vi "InitConfigParams.vi"(8 "error in (no error)":errorcluster, 10 "configuration file path":path, 11 "Camera in":refnum<class "CameraI2COUSB.lvclass">) -> (0 "error out":errorcluster, 3 "Camera out":refnum<class "CameraI2COUSB.lvclass">)   [LabVIEW 2020, in "CameraI2COUSB.lvlib" / "CameraI2COUSB.lvclass"]
uses:
  CameraI2COUSB.lvclass
  CameraI2COUSB.lvclass/CameraI2COUSB.ctl
  <vilib>/Utility/config.llb/Read Key (Path).vi
  <vilib>/Utility/config.llb/Read Key (String).vi
  <vilib>/Utility/config.llb/NI_LVConfig.lvlib
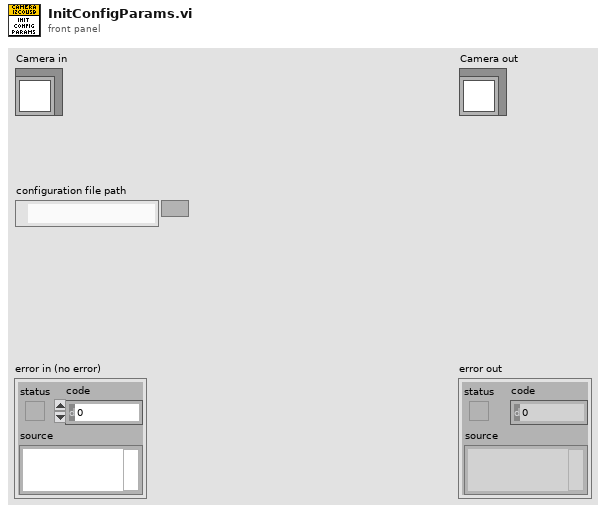
[diagram p1: front panel]
types:
  T1 = typedef "NI_LVConfig.lvlib/Config Data RefNum.ctl" = refnum<k1>
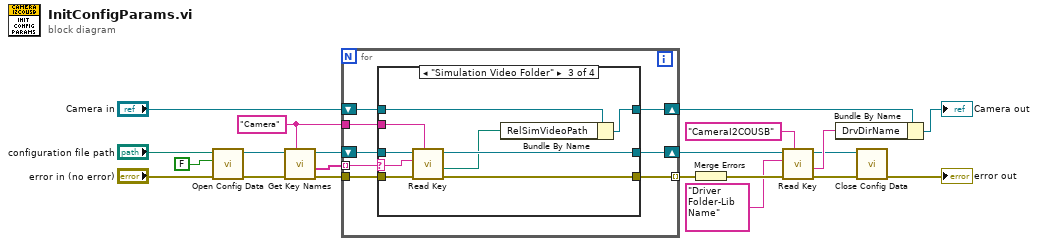
[diagram p0: block diagram]
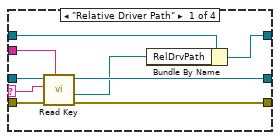
[diagram p2: hidden frame]
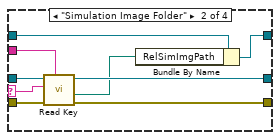
[diagram p3: hidden frame]
diagram:
  w14 = "Camera" ("section")
  n1 = call <vilib>:"Open Config Data.vi"("error in (no error)"="error in (no error)", "create file if necessary (T)"=FALSE, "configuration file path"="configuration file path") -> ("error out"=w21:errorcluster, "refnum"=w20:T1)  [unwired: 6 in, 1 out]
  n2 = call <vilib>:"Get Key Names.vi"("section"=w14, "error in (no error)"=w21, "refnum"=w20) -> ("error out"=w17:errorcluster, "key names"=w19:string[], "refnum out"=w18:T1)  [unwired: 5 in, 1 out]
  n3 = for {
    tunnel: w19 -> [w29] mode=indexing
    shift-right: [w25] -> w9
    shift-left: "Camera in" -> [w28]
    shift-right: [w24] -> w4
    shift-left: w18 -> [w27]
    tunnel: w17 -> [w26]
    tunnel: [w23] -> w16 mode=indexing
    tunnel: w14 -> [w22]
    n4 = case shown="\"Simulation Video Folder\"" w29 {
      selector: w29 -> [w36 w45 w54 _]
      tunnel: w28 -> [w35 w44 w53 w59]
      tunnel: w27 -> [w37 w46 w55 w58]
      tunnel: w26 -> [w38 w47 w56 w57]
      tunnel: [w34 w43 w52 w59] -> w25
      tunnel: [w33 w42 w51 w58] -> w24
      tunnel: [w32 w41 w50 w57] -> w23
      tunnel: w22 -> [w30 w39 w48 _]
      frame "Relative Driver Path" {
        n5 = call-poly <vilib>:"Read Key.vi"("section"=w30, "error in (no error)"=w38, "key"=w36, "refnum"=w37) -> ("error out"=w32:errorcluster, "value"=w31:path, "refnum out"=w33:T1)  [unwired: 4 in, 1 out]
        n6 = Bundle By Name(cluster=w35, "RelDrvPath"=w31) -> (w34:refnum<class "CameraI2COUSB.lvclass">)
      }
      frame "Simulation Image Folder" {
        n7 = call-poly <vilib>:"Read Key.vi"("section"=w39, "error in (no error)"=w47, "key"=w45, "refnum"=w46) -> ("error out"=w41:errorcluster, "value"=w40:path, "refnum out"=w42:T1)  [unwired: 4 in, 1 out]
        n8 = Bundle By Name(cluster=w44, "RelSimImgPath"=w40) -> (w43:refnum<class "CameraI2COUSB.lvclass">)
      }
      frame "Simulation Video Folder" {
        n9 = call-poly <vilib>:"Read Key.vi"("section"=w48, "error in (no error)"=w56, "key"=w54, "refnum"=w55) -> ("error out"=w50:errorcluster, "value"=w49:path, "refnum out"=w51:T1)  [unwired: 4 in, 1 out]
        n10 = Bundle By Name(cluster=w53, "RelSimVideoPath"=w49) -> (w52:refnum<class "CameraI2COUSB.lvclass">)
      }
      frame Default {
      }
    }
  }
  n11 = Merge Errors(w16) -> (w10:errorcluster)
  n12 = call-poly <vilib>:"Read Key.vi"("section"="CameraI2COUSB", "error in (no error)"=w10, "key"="Driver Folder-Lib Name", "refnum"=w4) -> ("error out"=w2:errorcluster, "value"=w6:string, "refnum out"=w3:T1)  [unwired: 4 in, 1 out]
  n13 = Bundle By Name(cluster=w9, "DrvDirName"=w6) -> (→"Camera out":refnum<class "CameraI2COUSB.lvclass">)
  n14 = call <vilib>:"Close Config Data.vi"("error in (no error)"=w2, "refnum"=w3) -> ("error out"=→"error out":errorcluster)  [unwired: 8 in, 1 out]
